vi "IVCurvePulsed2.vi"(10 "Program":string, 11 "UiDefinition":T3) -> (1 "appended array":dbl[][](array[numeric]), 3 "InfoCluster":T1)   [LabVIEW 2020]
uses:
  UIReferences.ctl
  D:/LabviewDXFViewer/LabviewDXFViewer/bin/Release/LabviewDXFViewer.exe
  LabviewDXFViewer/bin/Release/LabviewDXFViewer.exe
  CapacitanceInfos.ctl
  CapacitanceRecord.ctl
  Keithley 2600 Series/Keithley 2600 Series.lvlib
panel:
  out "error out 4":errorcluster
  out "error out 3":errorcluster
  out "error out 2":errorcluster
  out "error out":errorcluster
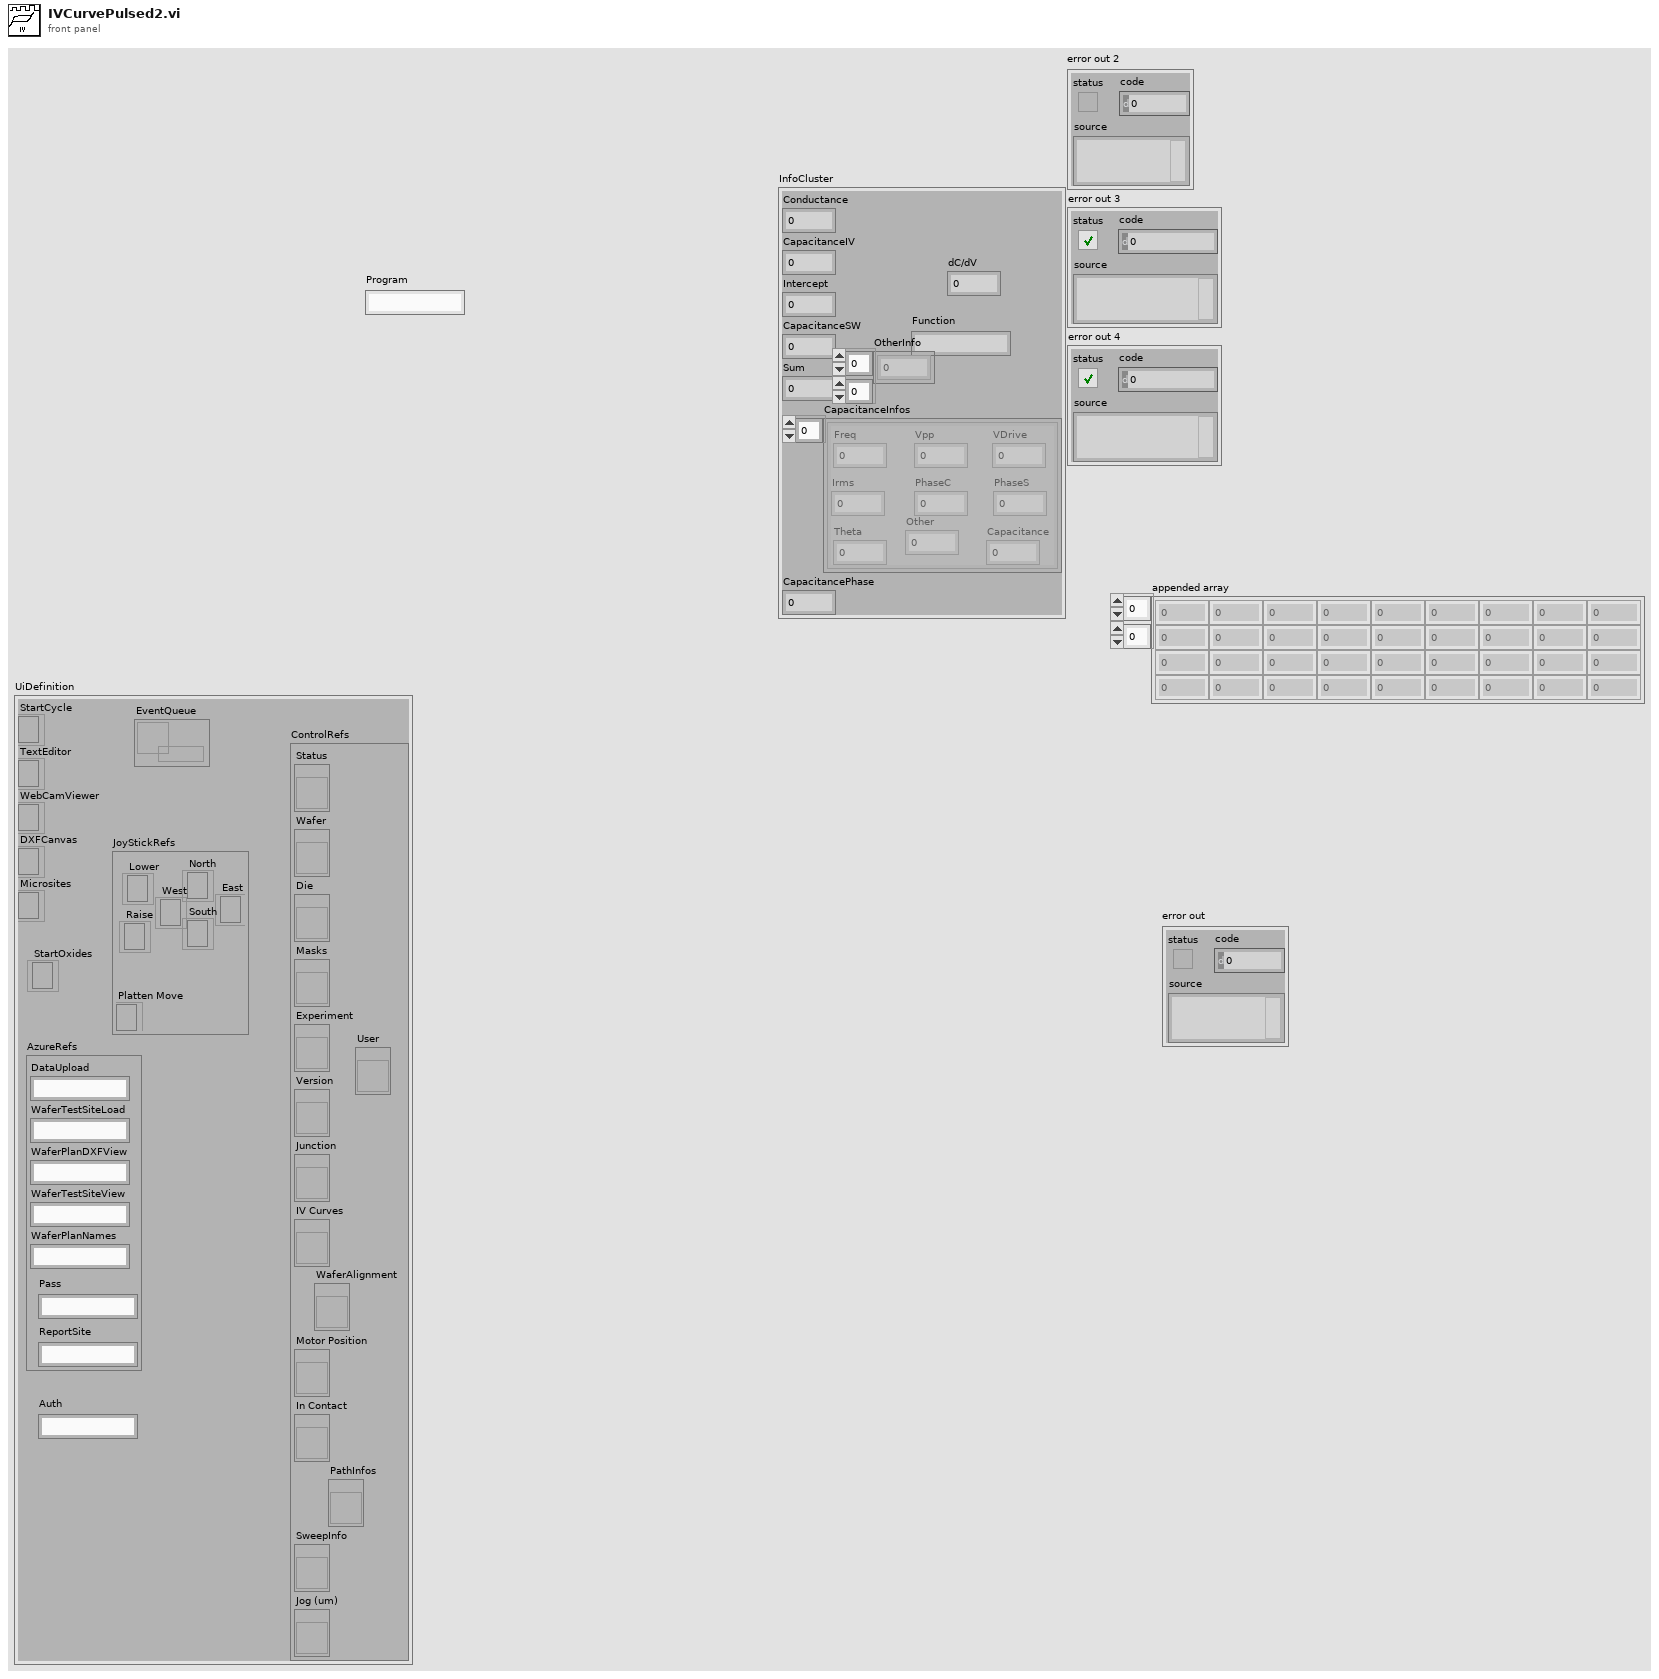
[diagram p1: front panel]
types:
  T1 = typedef "CapacitanceInfos.ctl" = cluster{"Conductance":dbl, "CapacitanceIV":dbl, "Intercept":dbl, "CapacitanceSW":dbl, "Sum":dbl, "CapacitanceInfos":T2[], "CapacitancePhase":dbl, "dC/dV":dbl, "Function":string, "OtherInfo":dbl[][]}
  T2 = typedef "CapacitanceRecord.ctl" = cluster{"Freq":dbl, "Vpp":dbl, "PhaseS":dbl, "Irms":dbl, "PhaseC":dbl, "Theta":dbl, "VDrive":dbl, "Capacitance":dbl, "Other":dbl}
  T3 = typedef "UIReferences.ctl" = cluster{"StartCycle":refnum<k24>, "TextEditor":refnum<k24>, "WebCamViewer":refnum<k24>, "DXFCanvas":refnum<k24>, "Microsites":refnum<k24>, "JoyStickRefs":cluster{"North":refnum<k24>, "Lower":refnum<k24>, "Raise":refnum<k24>, "Platten Move":refnum<k24>, "West":refnum<k24>, "East":refnum<k24>, "South":refnum<k24>}, "AzureRefs":cluster{"DataUpload":string, "WaferTestSiteLoad":string, "WaferPlanDXFView":string, "WaferTestSiteView":string, "WaferPlanNames":string, "Pass":string, "ReportSite":string}, "ControlRefs":cluster{"Status":refnum<vi>, "Wafer":refnum<vi>, "Die":refnum<vi>, "Masks":refnum<vi>, "Experiment":refnum<vi>, "Version":refnum<vi>, "Junction":refnum<vi>, "IV Curves":refnum<vi>, "Motor Position":refnum<vi>, "In Contact":refnum<vi>, "SweepInfo":refnum<vi>, "Jog (um)":refnum<vi>, "PathInfos":refnum<vi>, "User":refnum<vi>, "WaferAlignment":refnum<vi>}, "EventQueue":refnum<queue>, "StartOxides":refnum<k24>, "Auth":string}
  T4 = cluster{"Current Range":dbl, "Source Measure Unit Channel (0: Channel A)":i32, "Waveform":waveform(dbl), "VISA resource name":refnum<visa-resource-name>, "CodeText":string}
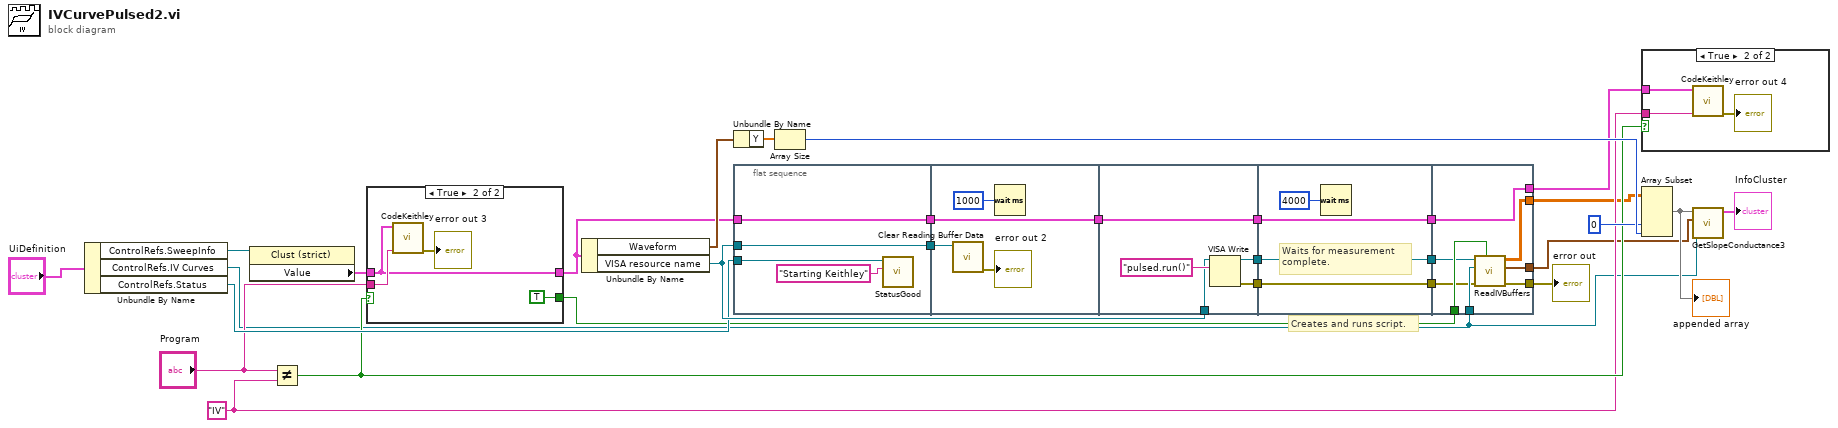
[diagram p0: block diagram]
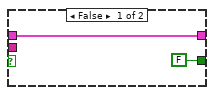
[diagram p3: hidden frame]
diagram:
  w10 = "IV" ("y")
  # "Creates and runs script."
  n1 = Unbundle By Name("UiDefinition") -> ("ControlRefs.SweepInfo"=w28:refnum<vi>, "ControlRefs.IV Curves"=w1:refnum<vi>, "ControlRefs.Status"=w20:refnum<vi>)
  n2 = property class="Clust (strict)"(reference=w28) -> ("Value"=w17:T4)  [unwired: 1 in, 2 out]
  n3 = Not Equal?(x="Program", y=w10) -> (x != y?=w11:bool)
  n4 = case shown="True" w11 {
    tunnel: [FALSE TRUE] -> w7
    tunnel: "Program" -> [_ w35]
    tunnel: w17 -> [w31 w34]
    tunnel: [w31 w34] -> w15
    frame False {
    }
    frame True {
      n5 = call "CodeKeithley.vi"("Program"=w35, "SweepInfo"=w34) -> ("error out"=→"error out 3":errorcluster)  [unwired: 9 in]
    }
  }
  n6 = Unbundle By Name(w15) -> ("Waveform"=w26:waveform(dbl), "VISA resource name"=w27:refnum<visa-resource-name>)
  n7 = Unbundle By Name(w26) -> ("Y"=w25:dbl[])
  n8 = flat-sequence {
    tunnel: w27 -> [w40]
    tunnel: [w40] -> w21
    tunnel: w20 -> [w39]
    tunnel: [w37] -> w16
    tunnel: w15 -> [w37]
    tunnel: w21 -> [w43]
    tunnel: w16 -> [w41]
    tunnel: [w41] -> w13
    tunnel: [w47] -> w30
    tunnel: w27 -> [w48]
    tunnel: [w46] -> w14
    tunnel: w13 -> [w46]
    tunnel: [w45] -> w2
    tunnel: w30 -> [w53]
    tunnel: w14 -> [w51]
    tunnel: [w53] -> w9
    tunnel: [w51] -> w8
    tunnel: [w50] -> w3
    tunnel: w2 -> [w50]
    tunnel: [w61] -> w12
    tunnel: w9 -> [w58]
    tunnel: w8 -> [w61]
    tunnel: w7 -> [w60]
    tunnel: w1 -> [w59]
    tunnel: [w57] -> w6
    tunnel: [w56] -> w5
    tunnel: [w55] -> w4
    tunnel: w3 -> [w54]
    frame #0 {
      n9 = call "StatusGood.vi"("Text.Text"="Starting Keithley", "String in"=w39) -> ()  [unwired: 10 in]
    }
    frame #1 {
      n10 = call "Clear Reading Buffer Data.vi"("VISA resource name"=w43) -> ("error out"=→"error out 2":errorcluster)  [unwired: 9 in, 1 out]
      n11 = Wait (ms)(milliseconds to wait=u32 1000) -> ()  [unwired: 1 out]
    }
    frame #2 {
      n12 = VISA Write(VISA resource name=w48, write buffer="pulsed.run()" ("format string")) -> (VISA resource name out=w47:refnum<visa-resource-name>, error out=w45:errorcluster)  [unwired: 1 in, 1 out]
    }
    frame #3 {
      # "Waits for measurement complete."
      n13 = Wait (ms)(milliseconds to wait=4000) -> ()  [unwired: 1 out]
    }
    frame #4 {
      n14 = call "ReadIVBuffers.vi"("GetCapacitors"=w60, "error in (no error)"=w54, "XYGraph Refnum"=w59, "VISA Refnum in"=w58) -> ("error out"=w57:errorcluster, "CapacitanceInfos"=w56:T2[], "Array"=w55:dbl[][])  [unwired: 5 in]
    }
  }
  n15 = Array Size(array=w25) -> (size(s)=w24:i32)
  n16 = case shown="True" w11 {
    tunnel: w10 -> [_ w64]
    tunnel: w12 -> [_ w63]
    frame False {
    }
    frame True {
      n17 = call "CodeKeithley.vi"("Program"=w64, "SweepInfo"=w63) -> ("error out"=→"error out 4":errorcluster)  [unwired: 9 in]
    }
  }
  n18 = Array Subset(array=w4, index (col)=0 ("index"), length (col)=w24) -> (w22:dbl[][])  [unwired: 2 in]
  "appended array" <- w22
  n19 = call "GetSlopeConductance3.vi"("XYGraph Refnum"=w1, "CapacitanceRecords"=w5, "Array in"=w22) -> ("InfoCluster"=→"InfoCluster":T1)  [unwired: 7 in, 1 out]
  "error out" <- w6
